vi "Contrast_adjust.vi"(6 "Basis":dbl, 7 "Swing voltage":dbl(slide)=2.0 scale=0.0..5.0, 8 "Auto adjust":bool, 9 "Color":i16, 10 "Pixel number":i32, 11 "Modulate date":dbl[](array[numeric])) -> (3 "Array":u32[](array[numeric]))   [LabVIEW 2016]
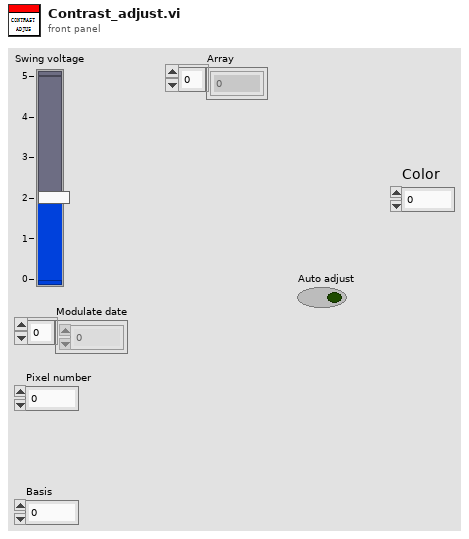
[diagram p1: front panel]
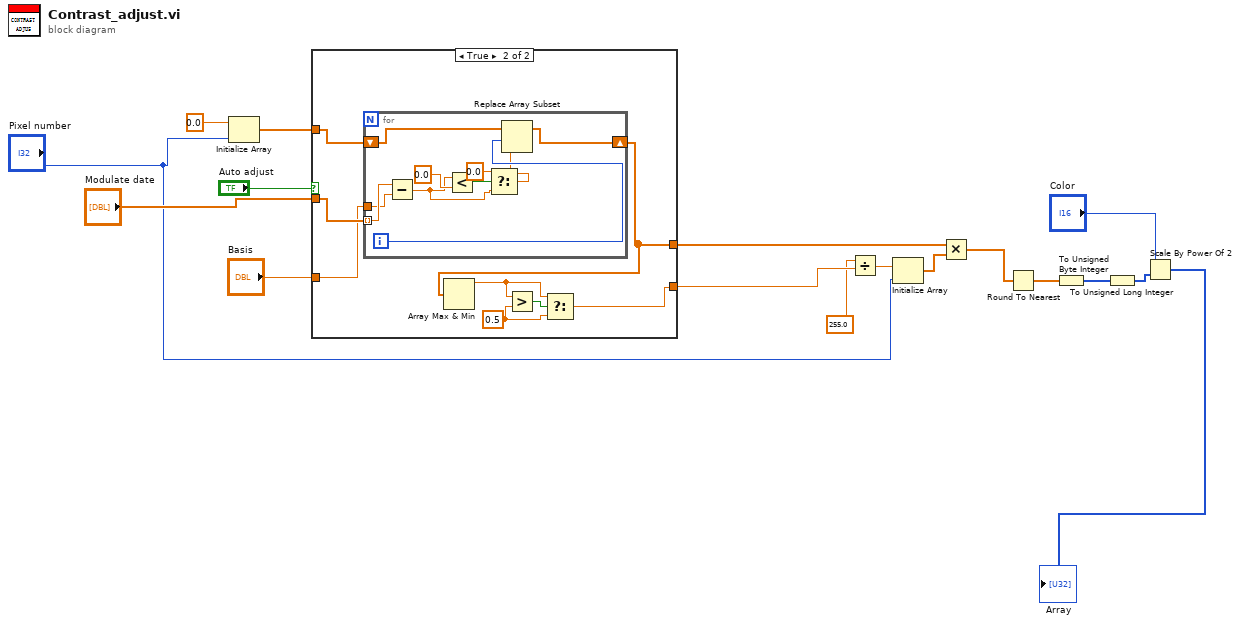
[diagram p0: block diagram]
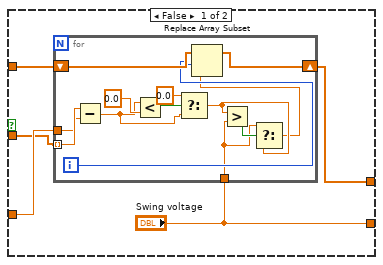
[diagram p2: hidden frame]
diagram:
  n1 = Initialize Array(0.0 ("element"), "Pixel number") -> (w13:dbl[])
  n2 = case shown="True" "Auto adjust" {
    tunnel: "Basis" -> [w22 w42]
    tunnel: "Modulate date" -> [w21 w43]
    tunnel: ["Swing voltage" w37] -> w15
    tunnel: [w19 w41] -> w14
    tunnel: w13 -> [w18 w36]
    frame False {
      n3 = for {
        shift-right: [w28] -> w19
        shift-left: w18 -> [w29]
        tunnel: "Swing voltage" -> [w25]
        tunnel: w21 -> [w24] mode=indexing
        tunnel: w22 -> [w23]
        i -> [w27]
        n4 = Subtract(x=w24, y=w23) -> (x-y=w32:dbl)
        n5 = Less?(x=w32, y=0.0) -> (x < y?=w34:bool)
        n6 = Select(t=0.0, s=w34, f=w32) -> (s? t:f=w30:dbl)
        n7 = Greater?(x=w30, y=w25) -> (0:w31:bool)
        n8 = Select(t=w25, s=w31, f=w30) -> (s? t:f=w26:dbl)
        n9 = Replace Array Subset(array=w29, new element=w26, index=w27) -> (w28:dbl[])
      }
    }
    frame True {
      w38 = 0.5 ("y")
      n10 = for {
        shift-right: [w49] -> w41
        shift-left: w36 -> [w44]
        tunnel: w43 -> [w47] mode=indexing
        tunnel: w42 -> [w46]
        i -> [w48]
        n11 = Subtract(x=w47, y=w46) -> (x-y=w50:dbl)
        n12 = Less?(x=w50, y=0.0) -> (x < y?=w52:bool)
        n13 = Select(t=0.0, s=w52, f=w50) -> (s? t:f=w45:dbl)
        n14 = Replace Array Subset(array=w44, new element=w45, index=w48) -> (w49:dbl[])
      }
      n15 = Array Max & Min(array=w41) -> (max value=w39:dbl)  [unwired: 3 out]
      n16 = Greater?(x=w39, y=w38) -> (0:w40:bool)
      n17 = Select(t=w39, s=w40, f=w38) -> (s? t:f=w37:dbl)
    }
  }
  n18 = Divide(x=255.0, y=w15) -> (x/y=w9:dbl)
  n19 = Initialize Array(w9, "Pixel number") -> (w10:dbl[])
  n20 = Multiply(x=w14, y=w10) -> (x*y=w11:dbl[])
  n21 = Round To Nearest(number=w11) -> (nearest integer value=w5:dbl[])
  n22 = To Unsigned Byte Integer(number=w5) -> (unsigned 8bit integer=w4:u8[])
  n23 = To Unsigned Long Integer(number=w4) -> (unsigned 32bit integer=w3:u32[])
  n24 = Scale By Power Of 2(n="Color", x=w3) -> (x*2^n=→"Array":u32[])
